vi "Result To String.vi"(11 "Result":refnum<vi>) -> (3 "SendCmd":string)   [LabVIEW 2019]
uses:
  Function/VisionSet/System/iVision/Controls/Parameter.ctl
  2f1d9a6e-04d9-4eca-a5af-4b65213a62f9.vi
  <vilib>/JDP Science/JSONtext/JSON text to Variant.vi
  <vilib>/vision/NI_Vision_Development_Module.lvlib
panel:
  out "OK":bool
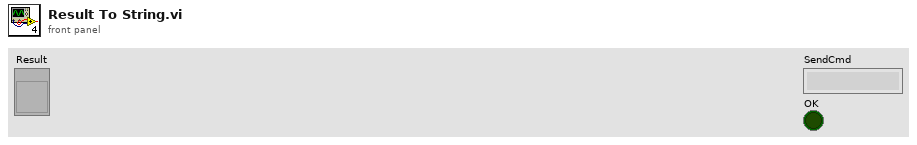
[diagram p1: front panel]
types:
  T1 = cluster{"ROI":string, "Numbers":i32, "Data":string[][]}[]
  T2 = cluster{"ROI":string, "Numbers":i32, "Data":string[][]}
  T3 = typedef "Parameter.ctl" = enum16{"Initialize", "Write", "Read", "WriteAll", "Save", "Load"}
  T4 = enum16{"Initial", "Write", "Read", "Save", "Load", "WrteAll"}
  T5 = typedef "ParameterData.ctl" = cluster{"Rotate Angle":dbl, "Rotate?":bool, "Calibration File Path":string, "Cal?":bool}
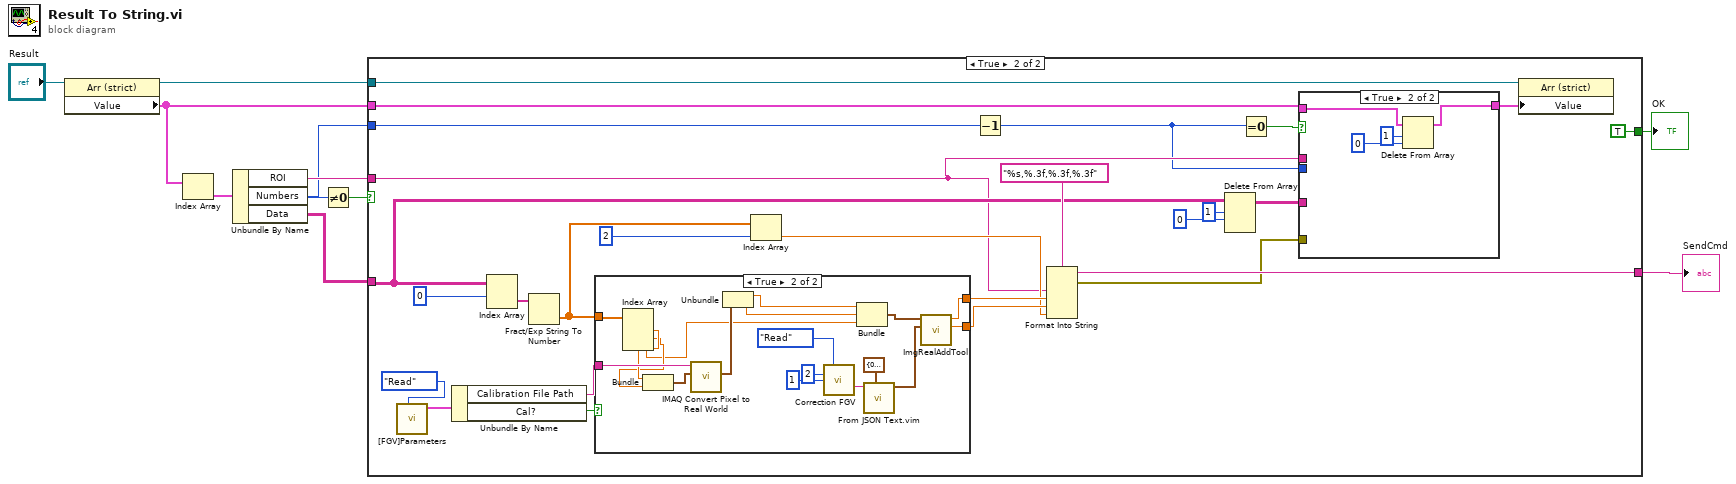
[diagram p0: block diagram]
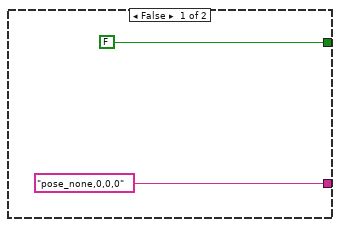
[diagram p2: hidden frame]
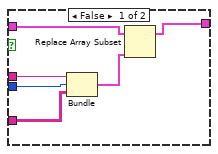
[diagram p3: hidden frame]
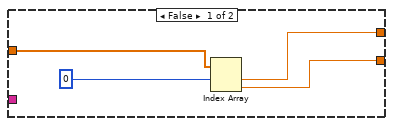
[diagram p4: hidden frame]
diagram:
  n1 = property class="Arr (strict)"(reference="Result") -> (reference out=w5:refnum<vi>, "Value"=w3:T1)  [unwired: 1 in, 1 out]
  n2 = Index Array(array=w3) -> (element=w10:T2)  [unwired: 1 in]
  n3 = Unbundle By Name(w10) -> ("ROI"=w7:string, "Numbers"=w4:i32, "Data"=w8:string[][])
  n4 = Not Equal To 0?(x=w4) -> (x != 0?=w9:bool)
  n5 = case shown="True" w9 {
    tunnel: w8 -> [_ w25]
    tunnel: w7 -> [_ w17]
    tunnel: ["pose_none,0,0,0" w27] -> w2
    tunnel: w5 -> [_ w22]
    tunnel: w4 -> [_ w26]
    tunnel: w3 -> [_ w20]
    tunnel: [FALSE TRUE] -> w1
    frame False {
    }
    frame True {
      n6 = call "[FGV]Parameters.vi"("Parameter"=Parameter."Read") -> ("ParameterData Out"=w30:T5)  [unwired: 9 in, 1 out]
      n7 = Unbundle By Name(w30) -> ("Calibration File Path"=w13:string, "Cal?"=w28:bool)
      n8 = Index Array(array=w25, index (row)=0) -> (element=w37:string[])  [unwired: 1 in]
      n9 = Fract/Exp String To Number(string=w37) -> (number=w36:dbl[])  [unwired: 3 in, 1 out]
      n10 = case shown="True" w28 {
        tunnel: w36 -> [w51 w62]
        tunnel: [w50 w64] -> w33
        tunnel: [w49 w63] -> w32
        tunnel: w13 -> [_ w61]
        frame False {
          n11 = Index Array(array=w51, index #1=0 ("index")) -> (element #1=w50:dbl, element #2=w49:dbl)  [unwired: 1 in]
        }
        frame True {
          n12 = Index Array(array=w62) -> (element #1=w60:dbl, element #2=w59:dbl, element #3=w54:dbl)  [unwired: 3 in]
          n13 = Bundle(w60, w59) -> (w58:cluster{dbl, dbl})  [unwired: 1 in]
          n14 = call "IMAQ Convert Pixel to Real World"("Pixel Coordinates"=w58, "Calibrated Image"=w61) -> ("Real World Coordinates"=w57:cluster{"X":sgl, "Y":sgl})  [unwired: 4 in, 5 out]
          n15 = Unbundle(w57) -> ("X"=w56:sgl, "Y"=w55:sgl)
          n16 = call "Correction FGV.vi"("Action"=T4."Read", "X"=2, "Y"=1) -> ("DataOut"=w70:string)  [unwired: 10 in, 2 out]
          n17 = Bundle("X"=w56, "Y"=w55, w54) -> (w53:cluster{"X":sgl, "Y":sgl, dbl})  [unwired: 1 in]
          n18 = call "From JSON Text.vim"("Data Type and Default Value"=cluster{"X":dbl, "Y":dbl, "Angle":dbl} {"X"=0.0, "Y"=0.0, "Angle"=0.0} ("ToolData"), "JSON"=w70) -> ("Data out"=w65:cluster{"X":dbl, "Y":dbl, "Angle":dbl})  [unwired: 8 in, 1 out]
          n19 = call "ImgRealAddTool.vi"("ToolData"=w65, "ImgRealData"=w53) -> ("YFinal"=w63:dbl, "XFinal"=w64:dbl)  [unwired: 8 in]
        }
      }
      n20 = Index Array(array=w36, index=2) -> (element=w31:dbl)
      n21 = Decrement(x=w26) -> (x-1=w16:i32)
      n22 = Format Into String(format string="%s,%.3f,%.3f,%.3f", w17, w33, w32, w31) -> (resulting string=w27:string, error out=w18:errorcluster)  [unwired: 2 in]
      n23 = Delete From Array(array=w25, length=1, index (row)=0) -> (array with subset deleted=w15:string[][])  [unwired: 1 in, 1 out]
      n24 = Equal To 0?(x=w16) -> (x = 0?=w21:bool)
      n25 = case shown="True" w21 {
        tunnel: w20 -> [w43 w46]
        tunnel: [w44 w45] -> w19
        tunnel: w18 -> [_ _]
        tunnel: w17 -> [w42 _]
        tunnel: w16 -> [w41 _]
        tunnel: w15 -> [w40 _]
        frame False {
          n26 = Bundle("ROI"=w42, w41, "Data"=w40) -> (w39:cluster{"ROI":string, i32, "Data":string[][]})  [unwired: 1 in]
          n27 = Replace Array Subset(array=w43, new element=w39) -> (w44:T1)  [unwired: 1 in]
        }
        frame True {
          n28 = Delete From Array(array=w46, length=1, index=0 ("index (row)")) -> (array with subset deleted=w45:T1)  [unwired: 1 out]
        }
      }
      n29 = property class="Arr (strict)"(reference=w22, "Value"=w19) -> ()  [unwired: 1 in, 2 out]
    }
  }
  "SendCmd" <- w2
  "OK" <- w1
